vi "GetWireRef__slk_mt.vi"(8 "error in (no error)":errorcluster, 11 "vi refnum in":refnum<vi>) -> (0 "error out":errorcluster, 2 "not found?":bool, 3 "wire refnum out":refnum<vi>)   [LabVIEW 2010, in "Lazyboots Menu Tool.lvlib"]
doc: "Returns wire ref if found."
uses:
  Library/Lazyboots Menu Tool.lvlib
panel:
  # "GetWireRef__slk_mt.vi\nReturns wire ref if found.\n\nNOTICE -- YOU MUST LEAVE THIS NOTICE IN PLACE.\n\nCopyright (c) 2011, LIANG LIU Shawn.Liu.cn@gmail.com\nAll rights reserved.\n\nRedistribution and use in source and binary forms, with or without modification, are permitted provided that the following conditions are met:\n-Redistributions of source code must retain the above copyright notice, this list of conditions and the following disclaimer.\n-Redistributions in binary form must reproduce the above copyright notice, this list of conditions and the following disclaimer in the documentation and/or other materials provided with the distribution.\n-Neither the name of the eLp nor the names of its contributors may be used to endorse or promote products derived from this software without specific prior written permission.\n\nTHIS SOFTWARE IS PROVIDED BY THE COPYRIGHT HOLDERS AND CONTRIBUTORS \"AS IS\" AND ANY EXPRESS OR IMPLIED WARRANTIES, INCLUDING, BUT NOT LIMITED TO, THE IMPLIED WARRANTIES OF MERCHANTABILITY AND FITNESS FOR A PARTICULAR PURPOSE ARE DISCLAIMED. IN NO EVENT SHALL THE COPYRIGHT HOLDER OR CONTRIBUTORS BE LIABLE FOR ANY DIRECT, INDIRECT, INCIDENTAL, SPECIAL, EXEMPLARY, OR CONSEQUENTIAL DAMAGES (INCLUDING, BUT NOT LIMITED TO, PROCUREMENT OF SUBSTITUTE GOODS OR SERVICES; LOSS OF USE, DATA, OR PROFITS; OR BUSINESS INTERRUPTION) HOWEVER CAUSED AND ON ANY THEORY OF LIABILITY, WHETHER IN CONTRACT, STRICT LIABILITY, OR TORT (INCLUDING NEGLIGENCE OR OTHERWISE) ARISING IN ANY WAY OUT OF THE USE OF THIS SOFTWARE, EVEN IF ADVISED OF THE POSSIBILITY OF SUCH DAMAGE."
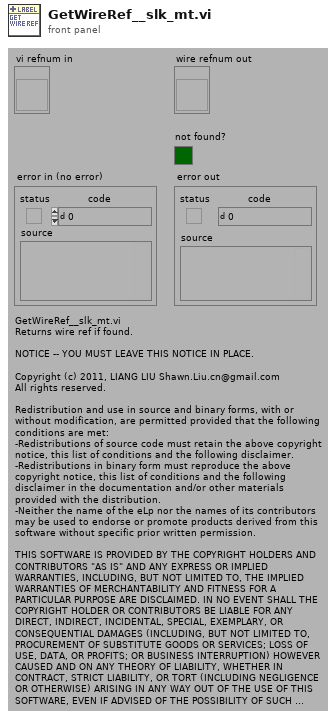
[diagram p1: front panel]
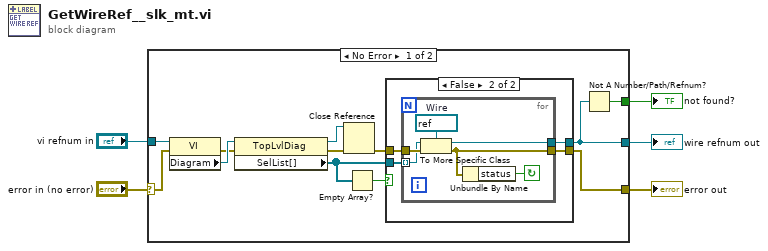
[diagram p0: block diagram]
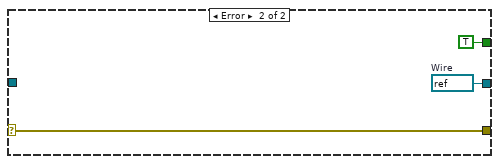
[diagram p3: hidden frame]
diagram:
  n1 = case shown="No Error" "error in (no error)" {
    selector: "error in (no error)" -> [w7 w31]
    tunnel: "vi refnum in" -> [w14 _]
    tunnel: [w9 TRUE] -> w4
    tunnel: [w8 w29] -> w3
    tunnel: [w6 w31] -> w1
    frame No Error {
      n2 = property on="Property Node" class="VI"(reference=w14, error in=w7) -> (error out=w15:errorcluster, "Diagram"=w17:refnum<vi>)  [unwired: 1 out]
      n3 = property on="Property Node" class="TopLvlDiag"(reference=w17, error in=w15) -> (reference out=w10:refnum<vi>, error out=w16:errorcluster, "SelList[]"=w13:refnum<vi>[])
      n4 = Close Reference(reference=w10, error in (no error)=w16) -> (error out=w11:errorcluster)
      n5 = Empty Array?(array=w13) -> (empty?=w12:bool)
      n6 = case shown="False" w12 {
        tunnel: w13 -> [_ w22]
        tunnel: w11 -> [w18 w21]
        tunnel: [w18 w20] -> w6
        tunnel: [_ w19] -> w8
        frame True {
        }
        frame False {
          n7 = for {
            tunnel: w22 -> [w23] mode=indexing
            tunnel: w21 -> [w27]
            tunnel: [w26] -> w20
            tunnel: [w24] -> w19
            stop <- w25 continue-if-true
            w28 = refnum<vi> refnum  # Wire
            n8 = To More Specific Class(target class=w28, reference=w23, error in=w27) -> (specific class reference=w24:refnum<vi>, error out=w26:errorcluster)
            n9 = Unbundle By Name(w26) -> ("status"=w25:bool)
          }
        }
      }
      n10 = Not A Number/Path/Refnum?(number/path/refnum=w8) -> (NaN/Path/Refnum?=w9:bool)
    }
    frame Error {
      w29 = refnum<vi> refnum  # Wire
    }
  }
  "wire refnum out" <- w3
  "not found?" <- w4
  "error out" <- w1
